vi "Serial Scope.vi"() -> ()   [LabVIEW 2015]
uses:
  <vilib>/Instr/_visa.llb/VISA Configure Serial Port (Instr).vi
panel:
  in  "Remplacer points par virgules":bool=TRUE
  in  "baud rate (9600)":u32=9600 caption="débit en bauds (9600)"
  in  "VISA resource name":refnum<visa-resource-name> caption="Nom de ressource VISA"
  in  "Mode trigger":enum16{"Auto", "Normal"}(ring)
  in  "Niveau trigger":dbl
  in  "Amplitude Maximum":dbl
  in  "Amplitude minimum":dbl
  in  "Nb échantillon":i32
  out "Graphe":dbl[][](graph)
  in  "Bouton Stop":bool
  # "Usage:\n- Les échantillons doivent être séparés par des nouvelles lignes.\n- Pour plus d'une courbe, séparez les échantillons par un espace.\n- Pour Windows français, activer le remplacement des points par virgules pour les données\n   en point flottant définies par des points."
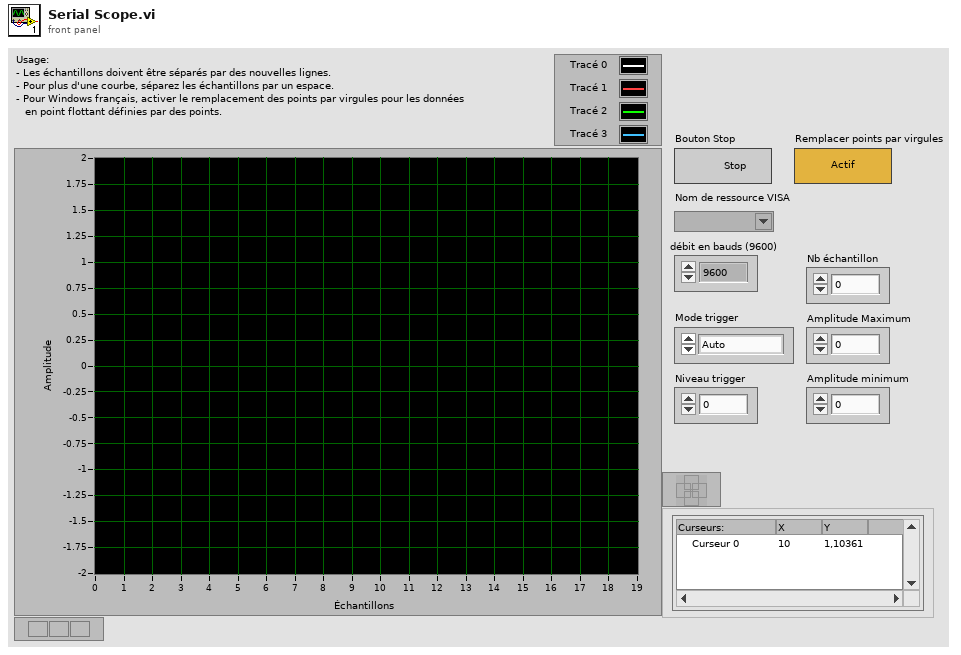
[diagram p1: front panel]
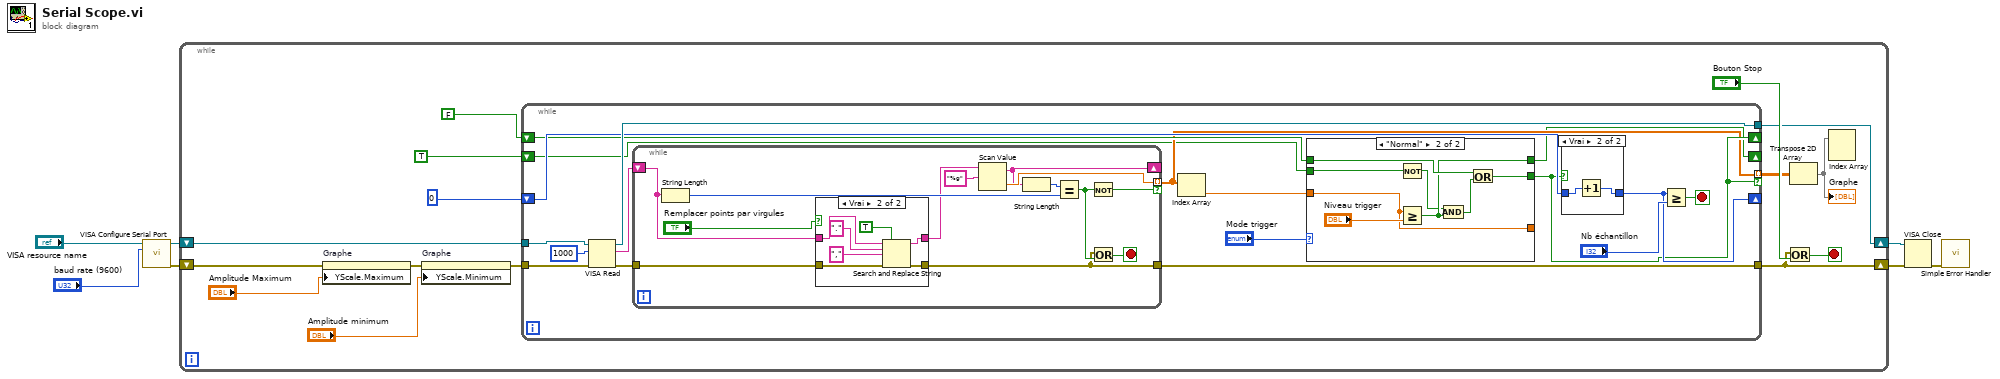
[diagram p0: block diagram]
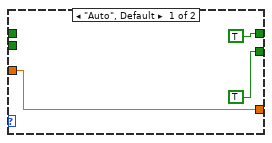
[diagram p3: hidden frame]
diagram:
  n1 = call-poly "VISA Configure Serial Port"("VISA resource name"="VISA resource name", "baud rate (9600)"="baud rate (9600)") -> ("VISA resource name out"=w7:refnum<visa-resource-name>, "error out"=w6:errorcluster)  [unwired: 12 in]
  n2 = while {
    shift-right: [w18] -> w5
    shift-left: w7 -> [w17]
    shift-right: [w19] -> w4
    shift-left: w6 -> [w9]
    stop <- w22 stop-if-true
    n3 = property on="Graphe" class="GraphWF (strict)"(error in=w9, "YScale.Maximum"="Amplitude Maximum") -> (error out=w10:errorcluster)  [unwired: 1 in, 1 out]
    n4 = property on="Graphe" class="GraphWF (strict)"(error in=w10, "YScale.Minimum"="Amplitude minimum") -> (error out=w8:errorcluster)  [unwired: 1 in, 1 out]
    n5 = while {
      tunnel: [w28] -> w20 mode=indexing if=w30
      tunnel: [w40] -> w18
      tunnel: [w23] -> w19
      tunnel: w8 -> [w39]
      tunnel: w17 -> [w38]
      shift-right: [w32] -> _
      shift-left: 0 -> [w33]
      shift-right: [w30] -> _
      shift-left: FALSE -> [w29]
      shift-right: [w25] -> _
      shift-left: TRUE -> [w26]
      stop <- w35 stop-if-true
      n6 = VISA Read(VISA resource name=w38, byte count=u32 1000 ("nombre d'octets"), error in (no error)=w39) -> (VISA resource name out=w40:refnum<visa-resource-name>, read buffer=w37:string, error out=w24:errorcluster)  [unwired: 1 out]
      n7 = while {
        shift-right: [w65] -> _
        shift-left: w37 -> [w61]
        tunnel: [w66] -> w28 mode=indexing if=w62
        tunnel: w24 -> [w59]
        tunnel: [w56] -> w23
        stop <- w57 stop-if-true
        n8 = String Length(string=w61) -> (length=w63:i32)
        n9 = case shown="Vrai" "Remplacer points par virgules" {
          tunnel: w61 -> [w68 w76]
          tunnel: [w68 w75] -> w60
          tunnel: w59 -> [w69 w72]
          tunnel: [w69 w71] -> w56
          frame False {
          }
          frame True {
            n10 = Search and Replace String(replace all?=TRUE ("tout remplacer ? (F)"), input string=w76, search string="." ("chaîne recherchée"), replace string="," ("chaîne de remplacement (\"\")"), error in=w72) -> (result string=w75:string, error out=w71:errorcluster)  [unwired: 3 in, 2 out]
          }
        }
        n11 = Scan Value(string=w60, format string="%g" ("chaîne de format")) -> (output string=w65:string, value=w66:dbl)  [unwired: 1 in]
        n12 = String Length(string=w65) -> (length=w64:i32)
        n13 = Equal?(x=w64, y=w63) -> (x = y?=w58:bool)
        n14 = Not(x=w58) -> (.not. x?=w62:bool)
        n15 = Or(x=w56, y=w58) -> (x .or. y?=w57:bool)
      }
      n16 = Index Array(array=w28) -> (element=w27:dbl)  [unwired: 1 in]
      n17 = case shown="\"Normal\"" "Mode trigger" {
        tunnel: [TRUE w54] -> w30
        tunnel: w29 -> [_ w53]
        tunnel: [w45 w50] -> _
        tunnel: w27 -> [w45 w50]
        tunnel: w26 -> [_ w48]
        tunnel: [TRUE w49] -> w25
        frame "Auto", Default {
        }
        frame "Normal" {
          n18 = Not(x=w48) -> (.not. x?=w47:bool)
          n19 = Greater Or Equal?(x=w50, y="Niveau trigger") -> (x >= y?=w49:bool)
          n20 = And(x=w47, y=w49) -> (x .and. y?=w51:bool)
          n21 = Or(x=w53, y=w51) -> (x .or. y?=w54:bool)
        }
      }
      n22 = case shown="Vrai" w30 {
        tunnel: w33 -> [w41 w43]
        tunnel: [w41 w42] -> w32
        frame False {
        }
        frame True {
          n23 = Increment(x=w43) -> (x+1=w42:i32)
        }
      }
      n24 = Greater Or Equal?(x=w32, y="Nb échantillon") -> (x >= y?=w35:bool)
    }
    n25 = Or(x=w19, y="Bouton Stop") -> (x .or. y?=w22:bool)
    n26 = Transpose 2D Array(2D array=w20) -> (transposed array=w16:dbl[][])
    "Graphe" <- w16
    n27 = Index Array(array=w16) -> ()  [unwired: 2 in, 1 out]
  }
  n28 = VISA Close(VISA resource name=w5, error in (no error)=w4) -> (error out=w3:errorcluster)
  n29 = call <vilib>:"Simple Error Handler.vi"("error in (no error)"=w3) -> ()  [unwired: 4 in, 5 out]
